vi "add_url_manually.vi"(6 "Volume URL in":string, 8 "error in (no error)":errorcluster, 9 "issue folder":path, 10 "manager_daemon":refnum<class "manager_daemon.lvclass">, 11 "Queue in":refnum<queue>) -> (0 "error out":errorcluster, 3 "Volume URL out":string)   [LabVIEW 2024, in "Download_Manager.lvlib"]
uses:
  Download_Manager.lvlib
  typedefs/job--cluster.ctl
  typedefs/job_type--enum.ctl
  comic_manager/manager_daemon/manager_daemon.lvclass
  WebScraper/series_class/series_class.lvclass
  WebScraper/series_class/series_class.lvclass/series_class.ctl
  WebScraper/comic_class/comic_class.lvclass
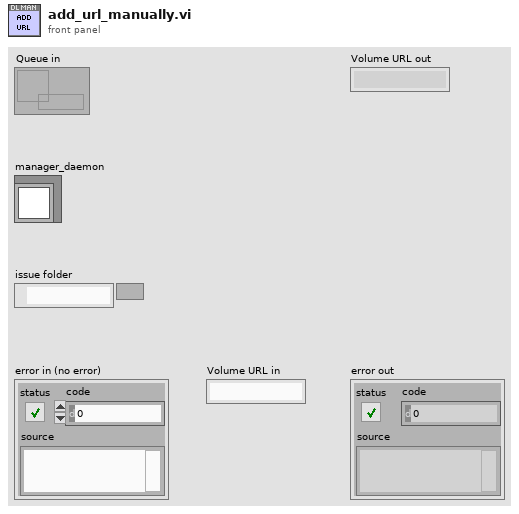
[diagram p1: front panel]
types:
  T1 = typedef "Download_Manager.lvlib/job_type--enum.ctl" = enum16{"check volume date", "check issues date", "download volume", "download isssue"}
  T2 = typedef "Download_Manager.lvlib/job--cluster.ctl" = cluster{"job type":T1, "job path":path, "id":i32, "url":string, "last updated":timestamp, "offset":i32, "original path":path}
  T3 = typedef "comic_class.lvclass/issueInfo--cluster.ctl" = cluster{"cover date":timestamp, "release date":timestamp, "number":string, "url":string, "small cover url":string, "name":string, "large cover url":string, "id":string, "creators":T4[], "characters":T5[], "teams":T6[], "locations":T7[], "concepts":T8[], "objects":T9[], "storyArcs":T10[], "description":string}
  T4 = typedef "comic_class.lvclass/creator--cluster.ctl" = cluster{"name":string, "role":string, "url":string}
  T5 = typedef "comic_class.lvclass/character--cluster.ctl" = cluster{"name":string, "url":string}
  T6 = typedef "comic_class.lvclass/team--cluster.ctl" = cluster{"name":string, "url":string}
  T7 = typedef "comic_class.lvclass/location--cluster.ctl" = cluster{"name":string, "url":string}
  T8 = typedef "comic_class.lvclass/concept--cluster.ctl" = cluster{"name":string, "url":string}
  T9 = typedef "comic_class.lvclass/thing--cluster.ctl" = cluster{"name":string, "url":string}
  T10 = typedef "comic_class.lvclass/storyArc--cluster.ctl" = cluster{"name":string, "url":string}
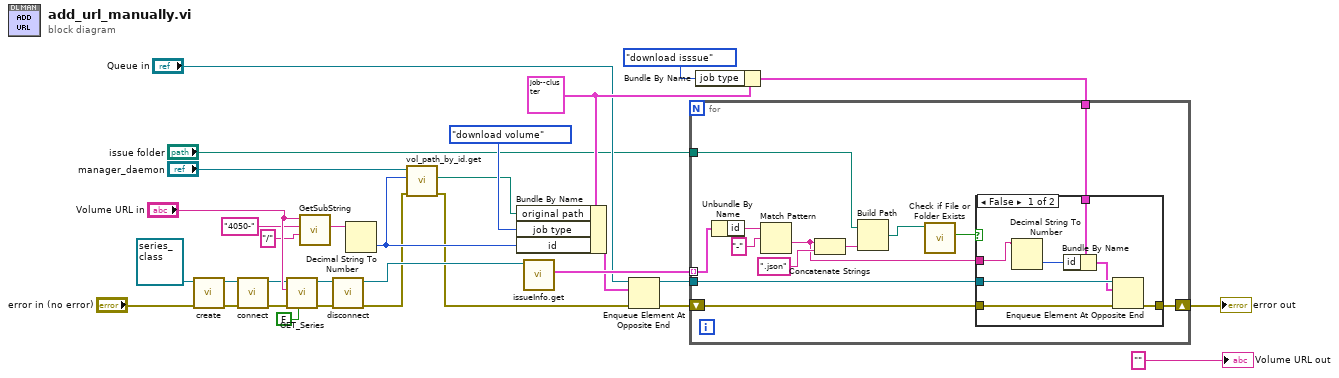
[diagram p0: block diagram]
diagram:
  w26 = T2 {"job type"=enum."check volume date", "job path"=path "", "id"=0, "url"="", "last updated"=timestamp(0 s since 1904-01-01), "offset"=0, "original path"=path ""} ("element")
  n1 = call "create.vi"("error in (no error)"="error in (no error)", "comic_class in"=refnum<class "series_class.lvclass"> refnum ("series_class.lvclass")) -> ("error out"=w11:errorcluster, "comic_class out"=w10:refnum<class "series_class.lvclass">)  [unwired: 8 in]
  n2 = call-dynamic "connect.vi"("error in (no error)"=w11, "comic_class in"=w10) -> ("error out"=w13:errorcluster, "comic_class out"=w12:refnum<class "series_class.lvclass">)  [unwired: 8 in]
  n3 = call "GET_Series.vi"("get all issues"=FALSE, "error in (no error)"=w13, "series URL"="Volume URL in", "ComicVine_class in"=w12) -> ("error out"=w15:errorcluster, "ComicVine_class out"=w16:refnum<class "series_class.lvclass">)  [unwired: 6 in]
  n4 = call "GetSubString.vi"("End Search"="/", "Start Search"="4050-" ("regular expression"), "String In"="Volume URL in") -> ("Match"=w20:string)  [unwired: 6 in, 2 out]
  n5 = call-dynamic "disconnect.vi"("error in (no error)"=w15, "comic_class in"=w16) -> ("error out"=w4:errorcluster, "comic_class out"=w18:refnum<class "series_class.lvclass">)  [unwired: 8 in]
  n6 = Decimal String To Number(string=w20) -> (number=w5:i32)  [unwired: 2 in, 1 out]
  n7 = call "vol_path_by_id.get.vi"("error in (no error)"=w4, "vol id"=w5, "manager_daemon"="manager_daemon") -> ("error out"=w3:errorcluster, "Path"=w2:path)  [unwired: 6 in, 1 out]
  n8 = Bundle By Name(cluster=w26, "original path"=w2, "job type"=job_type--enum."download volume", "id"=w5) -> (w22:T2)
  n9 = call "issueInfo.get.vi"("ComicVine_class in"=w18) -> ("issueInfo"=w24:T3[])  [unwired: 9 in, 1 out]
  n10 = Enqueue Element At Opposite End(queue="Queue in", element=w22, error in (no error)=w3) -> (queue out=w29:refnum<queue>, error out=w28:errorcluster)  [unwired: 1 in, 1 out]
  n11 = Bundle By Name(cluster=w26, "job type"=job_type--enum."download isssue") -> (w27:T2)
  n12 = for {
    tunnel: w24 -> [w44] mode=indexing
    tunnel: w27 -> [w43]
    shift-right: [w40] -> w30
    shift-left: w28 -> [w41]
    tunnel: w29 -> [w42]
    tunnel: "issue folder" -> [w35]
    n13 = Unbundle By Name(w44) -> ("id"=w39:string)
    n14 = Match Pattern(string=w39, regular expression="-") -> (after substring=w34:string)  [unwired: 1 in, 3 out]
    n15 = Concatenate Strings(w34, ".json" ("string")) -> (w36:string)
    n16 = Build Path(base path=w35, name or relative path=w36) -> (appended path=w33:path)
    n17 = call <vilib>:"Check if File or Folder Exists.vi"("path"=w33) -> ("file or folder exists?"=w32:bool)  [unwired: 8 in, 2 out]
    n18 = case shown="False" w32 {
      tunnel: w43 -> [w51 _]
      tunnel: w42 -> [w50 _]
      tunnel: w41 -> [w48 w52]
      tunnel: [w47 w52] -> w40
      tunnel: w34 -> [w45 _]
      frame False {
        n19 = Decimal String To Number(string=w45) -> (number=w46:i32)  [unwired: 2 in, 1 out]
        n20 = Bundle By Name(cluster=w51, "id"=w46) -> (w49:T2)
        n21 = Enqueue Element At Opposite End(queue=w50, element=w49, error in (no error)=w48) -> (error out=w47:errorcluster)  [unwired: 1 in, 2 out]
      }
      frame True {
      }
    }
  }
  "error out" <- w30
  "Volume URL out" <- "" ("Volume URL")
